vi "AVI视频回放.vi"() -> ()   [LabVIEW 2017]
panel:
  out "Elapsed Time (s)":dbl caption="已用时间(s)"
  in  "AVI Path":path
  out "Image":T1(plugin-control)
  in  "Stop":bool
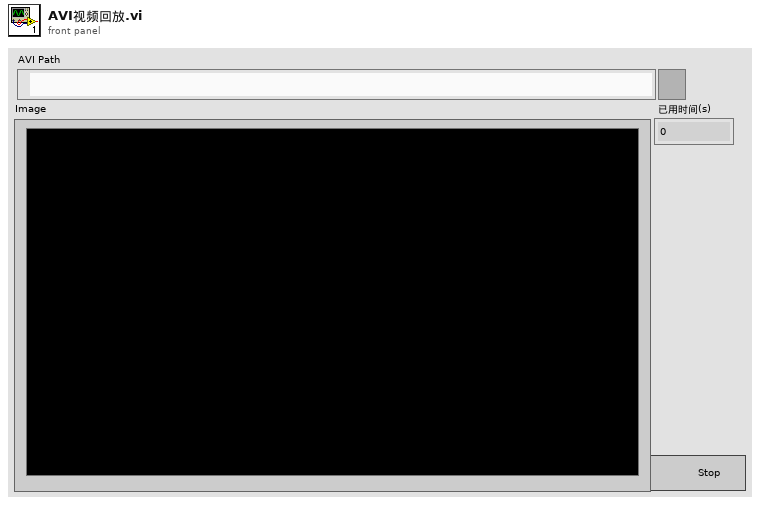
[diagram p1: front panel]
types:
  T1 = typedef "IMAQ Image.ctl" = refnum<image>
  T2 = typedef "AviRefnum.ctl" = refnum<k1>
  T3 = typedef "Image Type" = u32
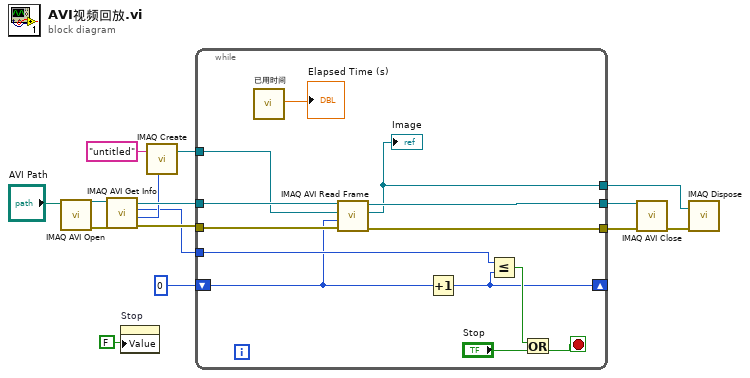
[diagram p0: block diagram]
diagram:
  n1 = call "IMAQ AVI Open"("AVI Path"="AVI Path") -> ("error out"=w8:errorcluster, "Avi Refnum"=w5:T2)  [unwired: 9 in]
  n2 = call "IMAQ AVI Get Info"("error in (no error)"=w8, "Avi Refnum"=w5) -> ("error out"=w7:errorcluster, "Image Type"=w4:T3, "Number of Frames"=w3:u32, "Avi Refnum (duplicate)"=w6:T2)  [unwired: 5 in, 1 out]
  n3 = property on="Stop" class="Bool (严格)"("Value"=FALSE ("Stop")) -> ()  [unwired: 2 in, 2 out]
  n4 = call "IMAQ Create"("Image Name"="untitled", "Image Type"=w4) -> ("New Image"=w10:T1)  [unwired: 3 in, 1 out]
  n5 = while {
    tunnel: [w24] -> w14
    tunnel: [w26] -> w13
    tunnel: w6 -> [w28]
    tunnel: w7 -> [w27]
    tunnel: [w25] -> w11
    tunnel: w10 -> [w23]
    tunnel: w3 -> [w21]
    shift-right: [w16] -> _
    shift-left: u32 0 -> [w20]
    stop <- w19 stop-if-true
    n6 = call "已用时间"() -> ("Elapsed Time (s)"=→"Elapsed Time (s)":dbl)  [unwired: 12 in, 7 out]
    n7 = call "IMAQ AVI Read Frame"("error in (no error)"=w27, "Frame Number"=w20, "Image"=w23, "Avi Refnum"=w28) -> ("error out"=w25:errorcluster, "Image Out"=w24:T1, "Avi Refnum (duplicate)"=w26:T2)  [unwired: 4 in, 1 out]
    "Image" <- w24
    n8 = Increment(x=w20) -> (x+1=w16:u32)
    n9 = Less Or Equal?(x=w21, y=w16) -> (x <= y?=w18:bool)
    n10 = Or(x=w18, y="Stop") -> (x .or. y?=w19:bool)
  }
  n11 = call "IMAQ AVI Close"("error in (no error)"=w11, "Avi Refnum"=w13) -> ("error out"=w15:errorcluster)  [unwired: 9 in]
  n12 = call "IMAQ Dispose"("Image"=w14, "error in (no error)"=w15) -> ()  [unwired: 4 in, 1 out]
